vi "LabVIEW Task Manager.vi"() -> ()   [LabVIEW 2010]
doc: "Use this template to create an application that executes until you click the Stop button. Unlike the Single Loop Application VI that uses polling, this VI uses the Event Structure."
uses:
  Error Task_Manager/Error Task_Manager Class/Error Task Manager.lvclass
panel:
  in  "error in (no error)":errorcluster
  in  "Search Clones Up To":i32=100 min=0 step=1
  in  "Timeout (ms)":i32=2000
  in  "Globals?":bool=TRUE
  in  "vit & ctt":bool=TRUE
  in  "Exclude vi.lib?":bool=TRUE
  in  "vi":bool
  in  "ctl":bool=TRUE
  in  "Refresh":bool
  in  "App Instance:":u16(ring) items=["Default Application Instance", "Task Manager.lvproj:My Computer"]
  in  "Data Tree":string[](tree)=["Get File Extension.vi"]
  in  "Close Front Panel":bool
  in  "Toggle Pause":bool
  in  "Pause Source":string
  in  "Initialize":bool
  in  "Close Block Diagram":bool
  in  "Pause":bool
  in  "Resume":bool
  in  "Toggle ExecHilite":bool
  in  "Open Front Panel":bool
  in  "Open Block Diagram":bool
  in  "Abort":bool
  # "Filter"
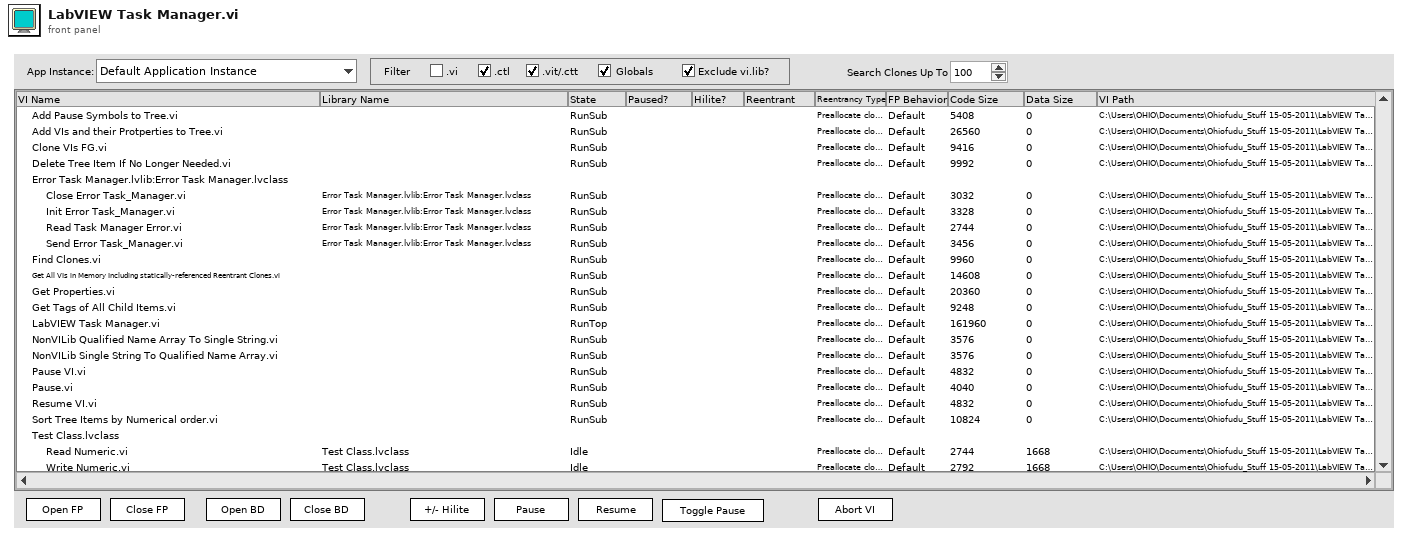
[diagram p1: front panel]
types:
  T1 = cluster{"Sort Column":i32, "Sorted AZ?":bool, "Data Tree Ref":refnum<vi>, "FP Ref":refnum<vi>, "Column Data Type":enum16{"String", "Numeric"}[], "AppInst":refnum<vi>}
  T2 = enum32{"Bad", "Idle", "Run top level", "Running"}
  T3 = typedef "LVPoint32TypeDef.ctl" = cluster{"Horizontal":i32, "Vertical":i32}
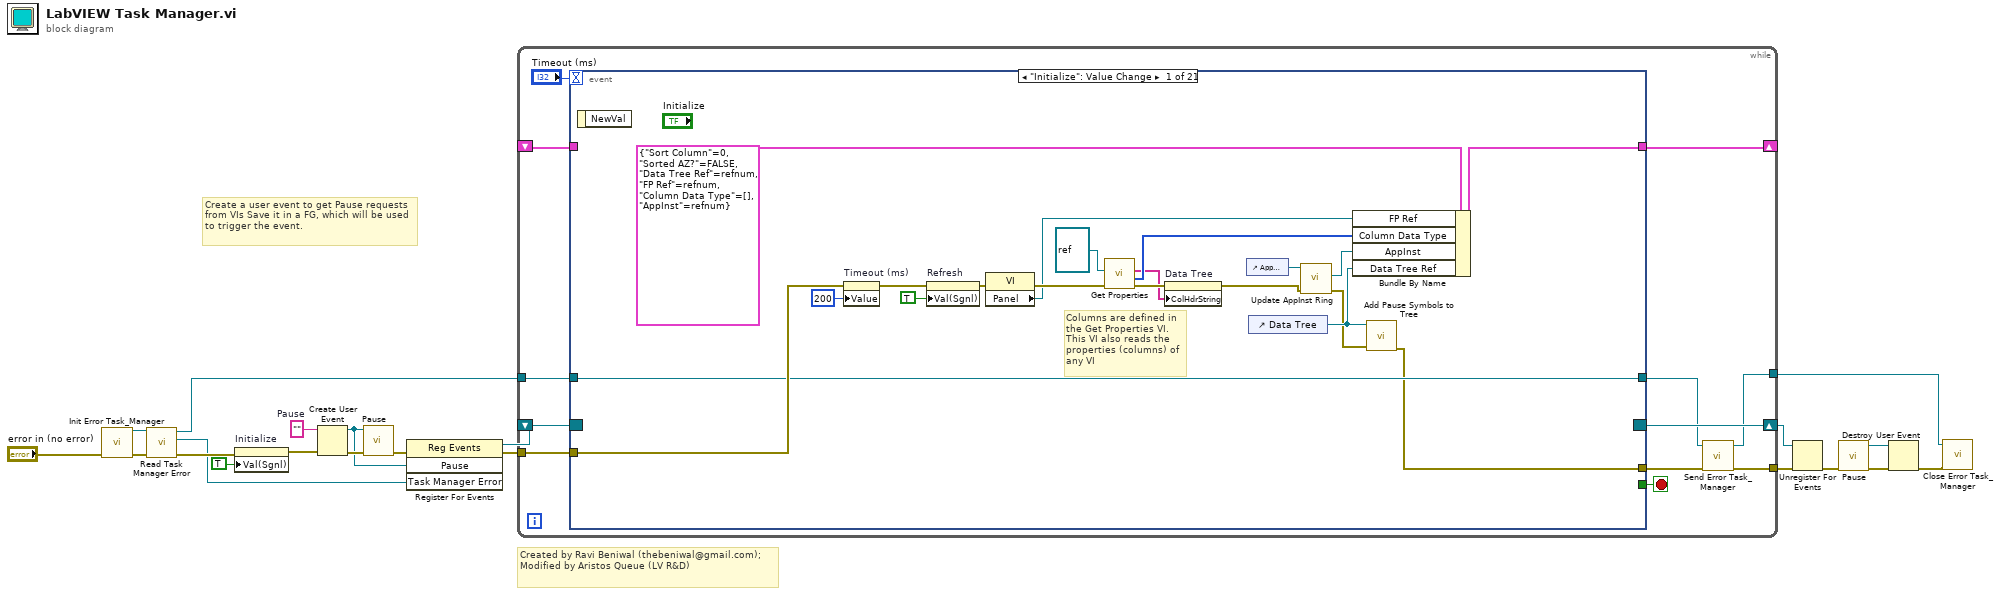
[diagram p0: block diagram]
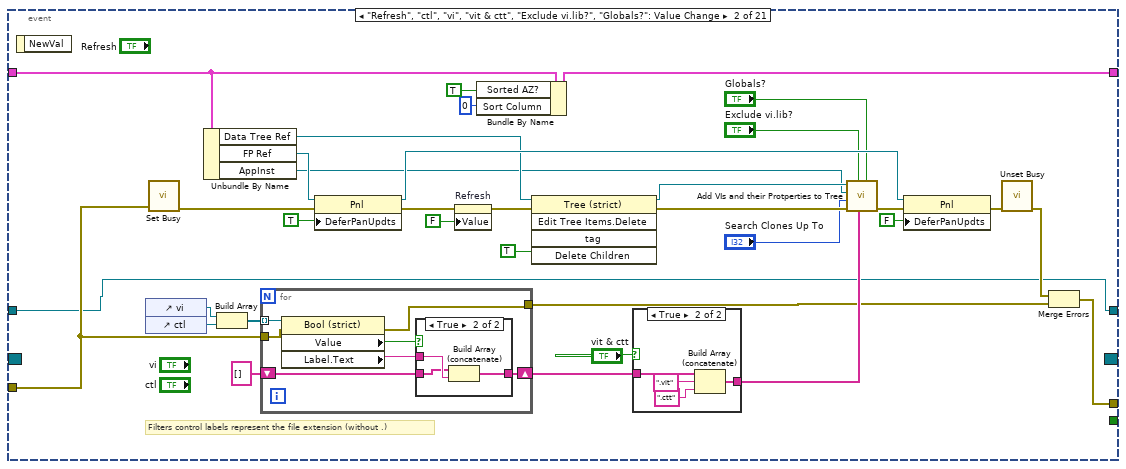
[diagram p2: hidden frame]
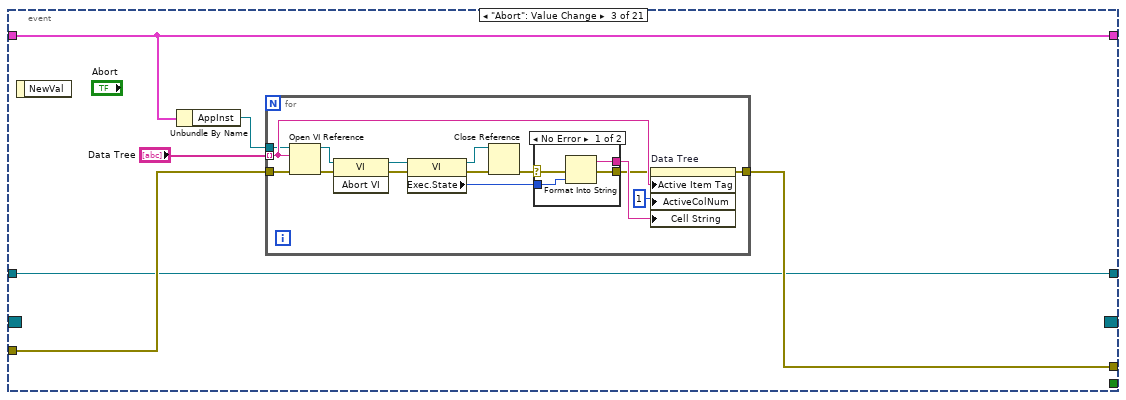
[diagram p5: hidden frame]
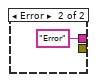
[diagram p6: hidden frame]
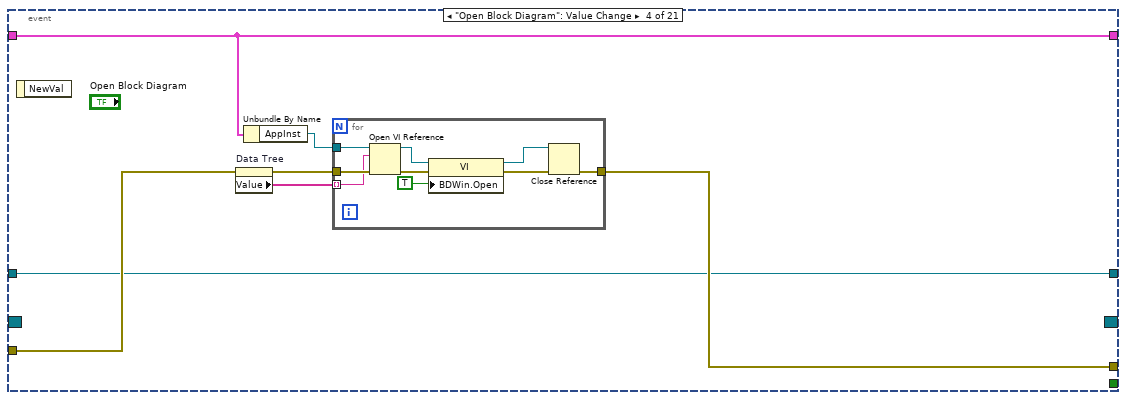
[diagram p7: hidden frame]
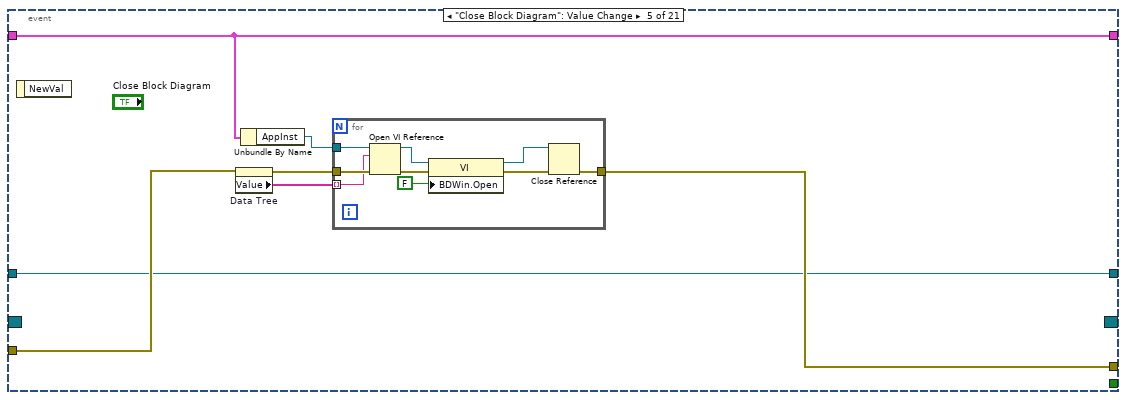
[diagram p8: hidden frame]
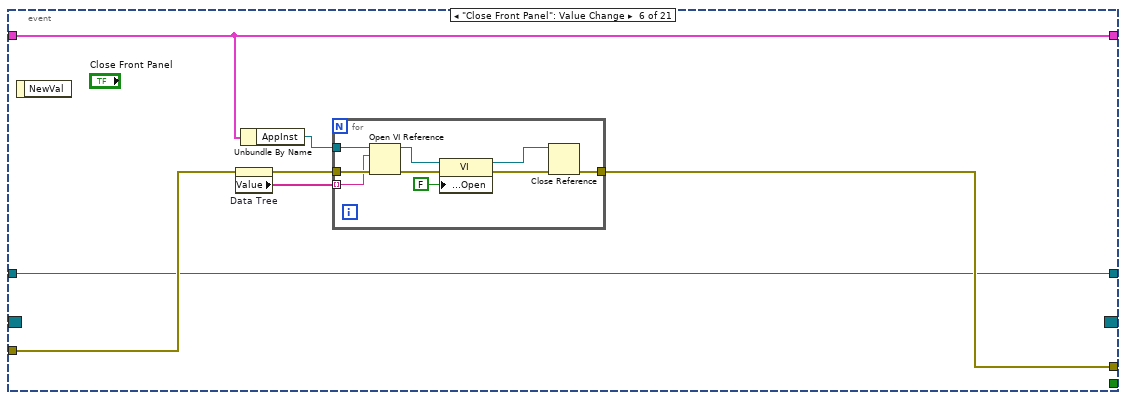
[diagram p9: hidden frame]
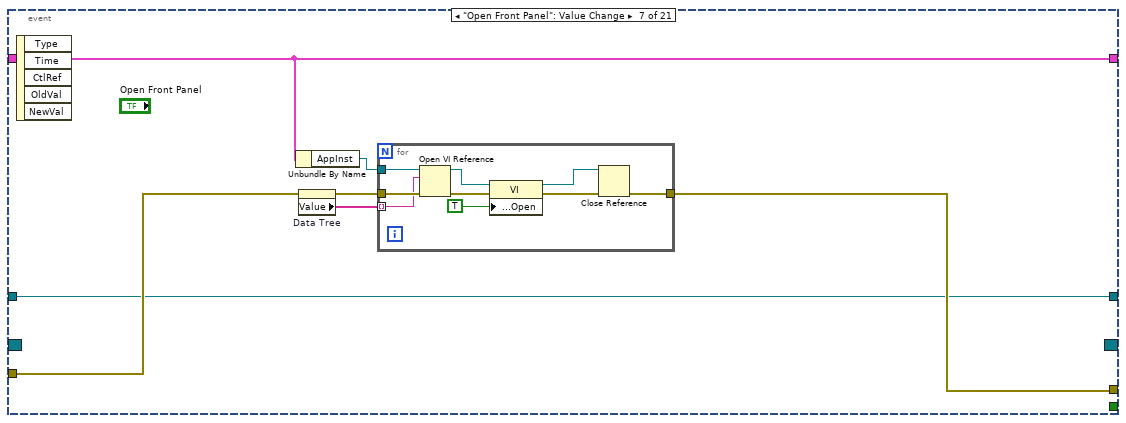
[diagram p10: hidden frame]
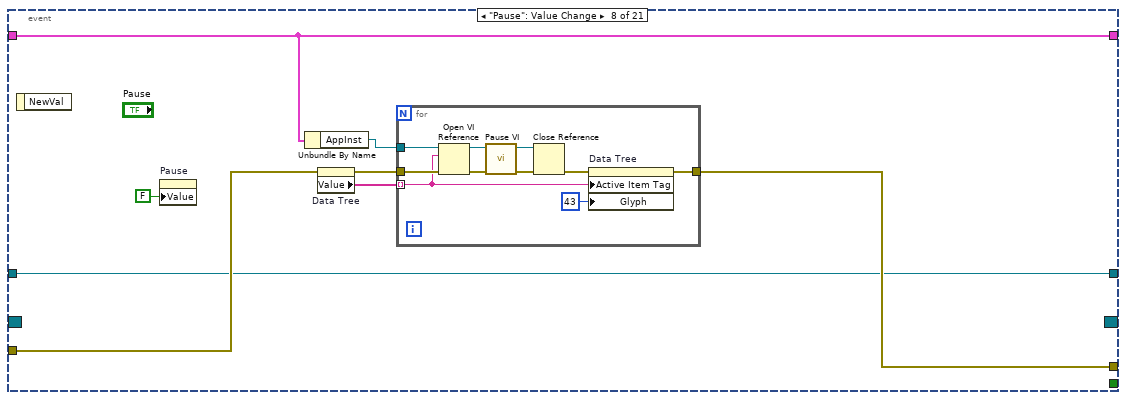
[diagram p11: hidden frame]
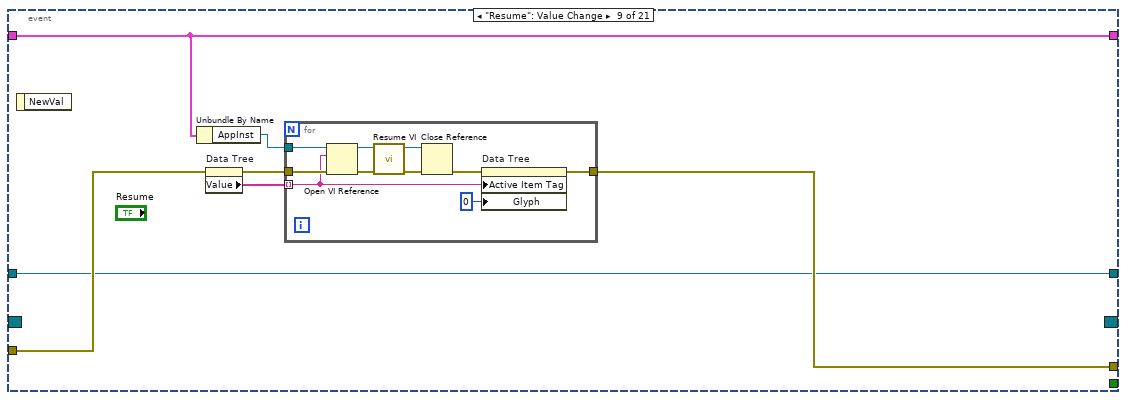
[diagram p12: hidden frame]
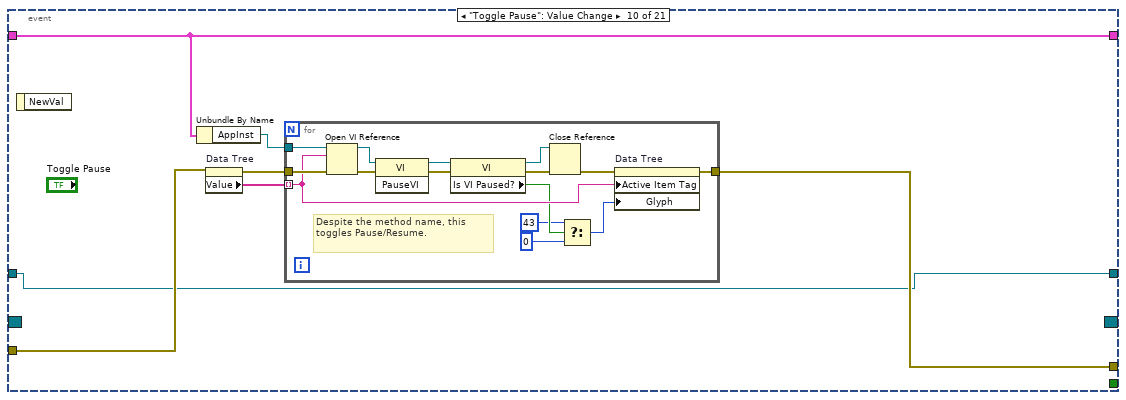
[diagram p13: hidden frame]
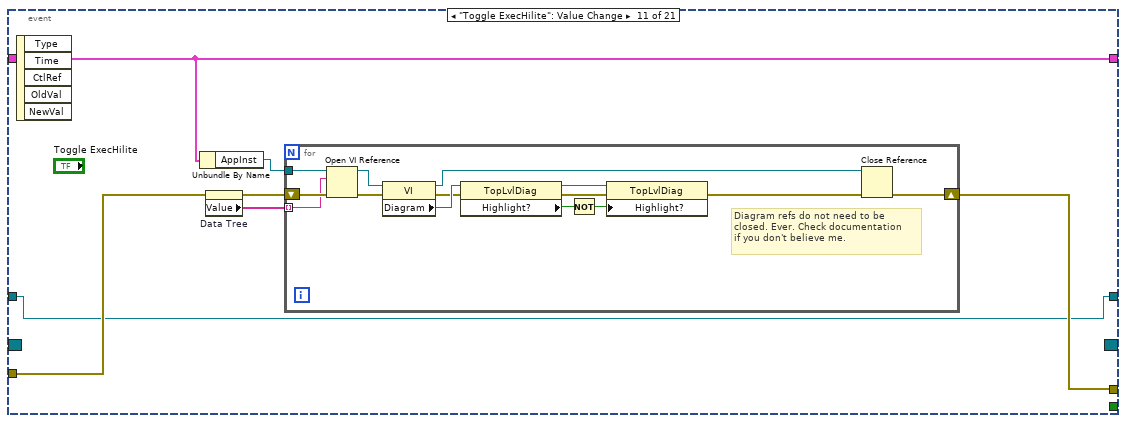
[diagram p14: hidden frame]
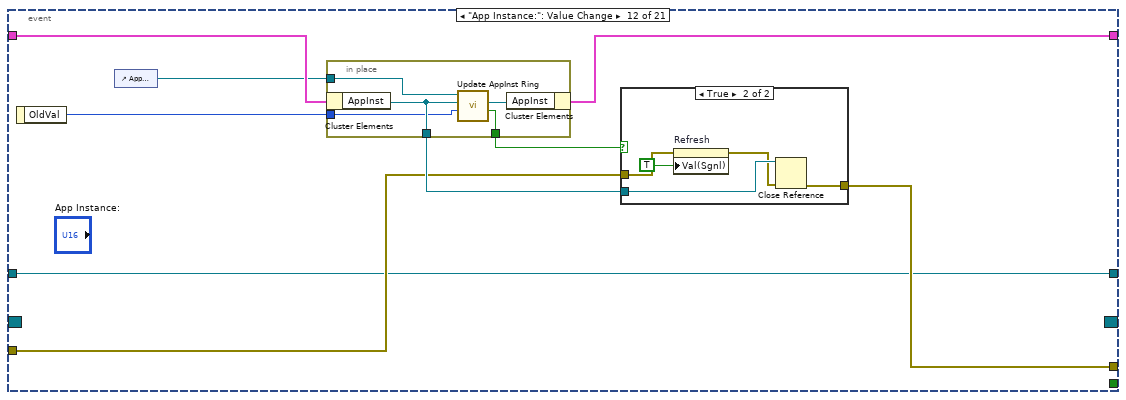
[diagram p15: hidden frame]
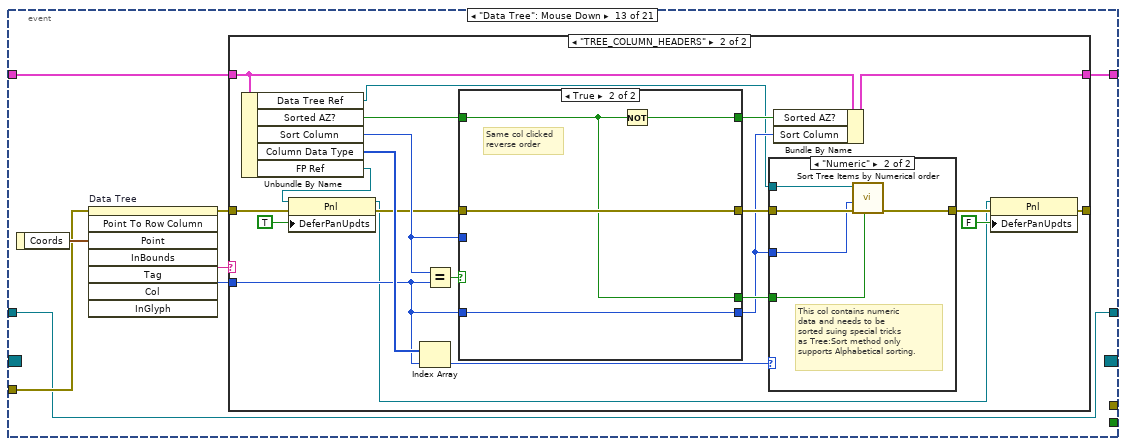
[diagram p17: hidden frame]
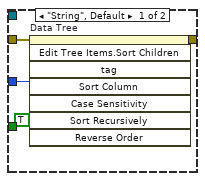
[diagram p19: hidden frame]
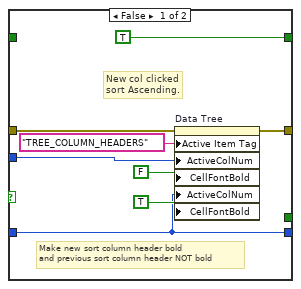
[diagram p20: hidden frame]
diagram:
  w14 = ""  # Pause
  # "Create a user event to get Pause requests from VIs Save it in a FG, which will be used to trigger the event."
  # "Created by Ravi Beniwal (thebeniwal@gmail.com);\nModified by Aristos Queue (LV R&D)"
  n1 = call "Init Error Task_Manager.vi"("error in (no error)"="error in (no error)") -> ("error out"=w6:errorcluster, "Error Task Manager out"=w7:refnum<class "Error Task Manager.lvclass">)  [unwired: 9 in]
  n2 = call "Read Task Manager Error.vi"("error in (no error)"=w6, "Error Task Manager in"=w7) -> ("error out"=w5:errorcluster, "Task Manager Error"=w4:refnum<user-event>, "Error Task Manager out"=w3:refnum<class "Error Task Manager.lvclass">)  [unwired: 7 in]
  n3 = property on="Initialize" class="Bool (strict)"(error in=w5, "Val(Sgnl)"=TRUE ("Value (Signaling)")) -> (error out=w9:errorcluster)  [unwired: 1 in, 1 out]
  n4 = Create User Event(user event datatype=w14, error in=w9) -> (user event=w12:refnum<user-event>, error out=w16:errorcluster)
  n5 = call "Pause.vi"("error in (no error)"=w16, "Pause user event"=w12) -> ("error out"=w15:errorcluster)  [unwired: 8 in, 1 out]
  n6 = register-events(error in=w15, w12, w4) -> (reference out=w13:refnum<event-registration>, error out=w11:errorcluster)  [unwired: 1 in]
  n7 = while {
    shift-right: [w30] -> _
    shift-left: _ -> [w31]
    shift-right: [w29] -> w20
    shift-left: w13 -> [w28]
    tunnel: w11 -> [w27]
    tunnel: [w23] -> w10
    tunnel: w3 -> [w26]
    tunnel: [w22] -> w1
    stop <- w33 stop-if-true
    n8 = event shown="[0] \"Initialize\": Value Change" {
      selector: w28 -> [_ _ _ _ _ _ _ _ _ _ _ _ _ _ _ _ _ _ _ _ _]
      dyn-events: [_ _ _ _ _ _ _ _ _ _ _ _ _ _ _ _ _ _ _ _ _] -> w29
      timeout: "Timeout (ms)" -> [_ _ _ _ _ _ _ _ _ _ _ _ _ _ _ _ _ _ _ _ _]
      tunnel: [_ _ _ _ _ _ _ _ _ _ _ _ _ _ TRUE ("stop") _ w417 _ _ w492 _] -> w33
      tunnel: w31 -> [_ w70 w108 w134 w149 w165 w181 w198 w215 w232 w254 w280 w294 w351 w397 w407 w419 w443 w489 w499 w511]
      tunnel: [w42 w73 w108 w134 w149 w165 w181 w198 w215 w232 w254 w279 w295 w351 w397 w407 w419 w443 w489 w499 w511] -> w30
      tunnel: w27 -> [w38 w58 w106 w132 w148 w164 w180 w196 w214 w231 w253 w274 w293 w347 w396 w402 w416 w430 w486 w491 w504]
      tunnel: [w34 w55 w105 w131 w147 w163 w179 w195 w213 w230 w252 w273 _ w346 w396 w401 w416 w429 w485 w491 w503] -> w24
      tunnel: w26 -> [w35 w54 w104 w130 w146 w162 w178 w194 w212 w229 w251 w272 w292 w345 w395 w400 w415 w428 w484 w490 w502]
      tunnel: [w35 w54 w104 w130 w146 w162 w178 w194 w212 w229 w251 w272 w292 w345 w395 w400 w415 w428 w484 w490 w502] -> w25
      event "Initialize": Value Change {
        # "Columns are defined in the Get Properties VI. This VI also reads the properties (columns) of any VI"
        n9 = event-data() -> ()  [unwired: 2 out]
        n10 = property on="Timeout (ms)" class="DigNum (strict)"(error in=w38, "Value"=200 ("Timeout (ms)")) -> (error out=w40:errorcluster)  [unwired: 1 in, 1 out]
        n11 = property on="Refresh" class="Bool (strict)"(error in=w40, "Val(Sgnl)"=TRUE ("Value (Signaling)")) -> (error out=w48:errorcluster)  [unwired: 1 in, 1 out]
        n12 = property class="VI"(error in=w48) -> (error out=w49:errorcluster, "Panel"=w47:refnum<vi>)  [unwired: 1 in, 1 out]
        n13 = call "Get Properties.vi"("error in"=w49, "AppInst"=refnum<vi> refnum) -> ("error out"=w46:errorcluster, "Column Data Type"=w50:enum16{"String", "Numeric"}[], "Column Labels"=w45:string[])  [unwired: 4 in, 3 out]
        n14 = property on="Data Tree" class="Tree (strict)"(error in=w46, "ColHdrString"=w45) -> (error out=w37:errorcluster)  [unwired: 1 in, 1 out]
        n15 = control-ref of="App Instance:"() -> (w51:refnum<vi>)
        n16 = control-ref of="Data Tree"() -> (w39:refnum<vi>)
        n17 = call "Update AppInst Ring.vi"("error in (no error)"=w37, "Ring in"=w51) -> ("error out"=w36:errorcluster, "AppInst out"=w52:refnum<vi>)  [unwired: 7 in, 1 out]
        n18 = Bundle By Name(cluster=T1 {"Sort Column"=0, "Sorted AZ?"=FALSE, "Data Tree Ref"=refnum, "FP Ref"=refnum, "Column Data Type"=[], "AppInst"=refnum}, "FP Ref"=w47, "Column Data Type"=w50, "AppInst"=w52, "Data Tree Ref"=w39) -> (w42:T1)
        n19 = call "Add Pause Symbols to Tree.vi"("error in"=w36, "Data Tree Ref"=w39) -> ("error out"=w34:errorcluster)  [unwired: 9 in]
      }
      event "Refresh", "ctl", "vi", "vit & ctt", "Exclude vi.lib?", "Globals?": Value Change {
        # "Filters control labels represent the file extension (without .)"
        n20 = event-data() -> ()  [unwired: 2 out]
        n21 = control-ref of="vi"() -> (w78:refnum<vi>)
        n22 = control-ref of="ctl"() -> (w65:refnum<vi>)
        n23 = call <vilib>:"Set Busy.vi"("error in (no error)"=w58) -> ("error out"=w67:errorcluster)  [unwired: 9 in, 1 out]
        n24 = Unbundle By Name(w70) -> ("Data Tree Ref"=w69:refnum<vi>, "FP Ref"=w68:refnum<vi>, "AppInst"=w60:refnum<vi>)
        n25 = Build Array(w78, w65) -> (w77:refnum<vi>[])
        n26 = for {
          tunnel: w77 -> [w99] mode=indexing
          shift-right: [w95] -> w64
          shift-left: string[] [] -> [w96]
          tunnel: w58 -> [w94]
          tunnel: [w93] -> w57
          n27 = property class="Bool (strict)"(reference=w99, error in=w94) -> (error out=w93:errorcluster, "Value"=w98:bool, "Label.Text"=w97:string)  [unwired: 1 out]
          n28 = case shown="True" w98 {
            tunnel: w97 -> [_ w103]
            tunnel: w96 -> [w100 w102]
            tunnel: [w100 w101] -> w95
            frame False {
            }
            frame True {
              n29 = Build Array (concatenate)(w102, w103) -> (w101:string[])
            }
          }
        }
        n30 = property class="Pnl"(reference=w68, error in=w67, "DeferPanUpdts"=TRUE ("Defer Panel Updates")) -> (reference out=w71:refnum<vi>, error out=w80:errorcluster)
        n31 = property on="Refresh" class="Bool (strict)"(error in=w80, "Value"=FALSE ("Refresh")) -> (error out=w84:errorcluster)  [unwired: 1 in, 1 out]
        n32 = Bundle By Name(cluster=w70, "Sorted AZ?"=TRUE, "Sort Column"=0) -> (w73:T1)
        n33 = invoke class="Tree (strict)" method="Edit Tree Items.Delete"(reference=w69, error in=w84, "Delete Children"=TRUE ("Delete Children?")) -> (reference out=w85:refnum<vi>, error out=w86:errorcluster)  [unwired: 2 in, 3 out]
        n34 = case shown="True" "vit & ctt" {
          tunnel: w64 -> [w88 w92]
          tunnel: [w88 w89] -> w62
          frame False {
          }
          frame True {
            n35 = Build Array (concatenate)(w92, ".vit", ".ctt") -> (w89:string[])
          }
        }
        n36 = call "Add VIs and their Protperties to Tree.vi"("Globals?"="Globals?", "File Extension Filters"=w62, "Exclude vi.lib?"="Exclude vi.lib?", "error in"=w86, "Search Clones Up To"="Search Clones Up To", "AppInst"=w60, "Data Tree"=w85) -> ("error out"=w72:errorcluster)  [unwired: 4 in]
        n37 = property class="Pnl"(reference=w71, error in=w72, "DeferPanUpdts"=FALSE ("Defer Panel Updates")) -> (error out=w79:errorcluster)  [unwired: 1 out]
        n38 = call <vilib>:"Unset Busy.vi"("error in (no error)"=w79) -> ("error out"=w56:errorcluster)  [unwired: 10 in]
        n39 = Merge Errors(w56, w57) -> (w55:errorcluster)
      }
      event "Abort": Value Change {
        n40 = event-data() -> ()  [unwired: 2 out]
        n41 = Unbundle By Name(w108) -> ("AppInst"=w107:refnum<vi>)
        n42 = for {
          tunnel: [w119] -> w105
          tunnel: "Data Tree" -> [w117] mode=indexing
          tunnel: w107 -> [w111]
          tunnel: w106 -> [w110]
          n43 = Open VI Reference(application reference (local)=w111, vi path=w117, error in (no error)=w110) -> (vi reference=w123:refnum<vi>, error out=w124:errorcluster)  [unwired: 3 out]
          n44 = invoke class="VI" method="Abort VI"(reference=w123, error in=w124) -> (reference out=w121:refnum<vi>, error out=w112:errorcluster)  [unwired: 1 in, 1 out]
          n45 = property class="VI"(reference=w121, error in=w112) -> (reference out=w120:refnum<vi>, error out=w115:errorcluster, "Exec.State"=w122:T2)
          n46 = Close Reference(reference=w120, error in (no error)=w115) -> (error out=w113:errorcluster)
          n47 = case shown="No Error" w113 {
            selector: w113 -> [w125 _]
            tunnel: w122 -> [w128 _]
            tunnel: [w127 "Error"] -> w118
            tunnel: [w126 _] -> w114
            frame No Error {
              n48 = Format Into String(error in=w125, w128) -> (resulting string=w127:string, error out=w126:errorcluster)  [unwired: 2 in]
            }
            frame Error {
            }
          }
          n49 = property on="Data Tree" class="Tree (strict)"(error in=w114, "Active Item Tag"=w117, "ActiveColNum"=1 ("Active Cell:Active Column Number"), "Cell String"=w118) -> (error out=w119:errorcluster)  [unwired: 1 in, 1 out]
        }
      }
      event "Open Block Diagram": Value Change {
        n50 = event-data() -> ()  [unwired: 2 out]
        n51 = property on="Data Tree" class="Tree (strict)"(error in=w132) -> (error out=w136:errorcluster, "Value"=w135:string[])  [unwired: 1 in, 1 out]
        n52 = Unbundle By Name(w134) -> ("AppInst"=w133:refnum<vi>)
        n53 = for {
          tunnel: [w145] -> w131
          tunnel: w136 -> [w144]
          tunnel: w135 -> [w143] mode=indexing
          tunnel: w133 -> [w137]
          n54 = Open VI Reference(application reference (local)=w137, vi path=w143, error in (no error)=w144) -> (vi reference=w141:refnum<vi>, error out=w142:errorcluster)  [unwired: 3 out]
          n55 = property class="VI"(reference=w141, error in=w142, "BDWin.Open"=TRUE ("Block Diagram Window:Open")) -> (reference out=w140:refnum<vi>, error out=w139:errorcluster)
          n56 = Close Reference(reference=w140, error in (no error)=w139) -> (error out=w145:errorcluster)
        }
      }
      event "Close Block Diagram": Value Change {
        n57 = event-data() -> ()  [unwired: 2 out]
        n58 = property on="Data Tree" class="Tree (strict)"(error in=w148) -> (error out=w152:errorcluster, "Value"=w151:string[])  [unwired: 1 in, 1 out]
        n59 = Unbundle By Name(w149) -> ("AppInst"=w150:refnum<vi>)
        n60 = for {
          tunnel: [w161] -> w147
          tunnel: w152 -> [w160]
          tunnel: w151 -> [w159] mode=indexing
          tunnel: w150 -> [w153]
          n61 = Open VI Reference(application reference (local)=w153, vi path=w159, error in (no error)=w160) -> (vi reference=w157:refnum<vi>, error out=w158:errorcluster)  [unwired: 3 out]
          n62 = property class="VI"(reference=w157, error in=w158, "BDWin.Open"=FALSE ("Block Diagram Window:Open")) -> (reference out=w156:refnum<vi>, error out=w155:errorcluster)
          n63 = Close Reference(reference=w156, error in (no error)=w155) -> (error out=w161:errorcluster)
        }
      }
      event "Close Front Panel": Value Change {
        n64 = event-data() -> ()  [unwired: 2 out]
        n65 = property on="Data Tree" class="Tree (strict)"(error in=w164) -> (error out=w168:errorcluster, "Value"=w167:string[])  [unwired: 1 in, 1 out]
        n66 = Unbundle By Name(w165) -> ("AppInst"=w166:refnum<vi>)
        n67 = for {
          tunnel: [w177] -> w163
          tunnel: w168 -> [w176]
          tunnel: w167 -> [w175] mode=indexing
          tunnel: w166 -> [w169]
          n68 = Open VI Reference(application reference (local)=w169, vi path=w175, error in (no error)=w176) -> (vi reference=w173:refnum<vi>, error out=w174:errorcluster)  [unwired: 3 out]
          n69 = property class="VI"(reference=w173, error in=w174, "Front Panel.Open"=FALSE ("Block Diagram Window:Open")) -> (reference out=w172:refnum<vi>, error out=w171:errorcluster)
          n70 = Close Reference(reference=w172, error in (no error)=w171) -> (error out=w177:errorcluster)
        }
      }
      event "Open Front Panel": Value Change {
        n71 = event-data() -> ()  [unwired: 6 out]
        n72 = Unbundle By Name(w181) -> ("AppInst"=w182:refnum<vi>)
        n73 = property on="Data Tree" class="Tree (strict)"(error in=w180) -> (error out=w184:errorcluster, "Value"=w183:string[])  [unwired: 1 in, 1 out]
        n74 = for {
          tunnel: [w193] -> w179
          tunnel: w184 -> [w192]
          tunnel: w183 -> [w191] mode=indexing
          tunnel: w182 -> [w185]
          n75 = Open VI Reference(application reference (local)=w185, vi path=w191, error in (no error)=w192) -> (vi reference=w189:refnum<vi>, error out=w190:errorcluster)  [unwired: 3 out]
          n76 = property class="VI"(reference=w189, error in=w190, "Front Panel.Open"=TRUE ("Block Diagram Window:Open")) -> (reference out=w188:refnum<vi>, error out=w187:errorcluster)
          n77 = Close Reference(reference=w188, error in (no error)=w187) -> (error out=w193:errorcluster)
        }
      }
      event "Pause": Value Change {
        n78 = event-data() -> ()  [unwired: 2 out]
        n79 = property on="Pause" class="Bool (strict)"("Value"=FALSE ("Pause")) -> ()  [unwired: 2 in, 2 out]
        n80 = Unbundle By Name(w198) -> ("AppInst"=w199:refnum<vi>)
        n81 = property on="Data Tree" class="Tree (strict)"(error in=w196) -> (error out=w200:errorcluster, "Value"=w201:string[])  [unwired: 1 in, 1 out]
        n82 = for {
          tunnel: w201 -> [w204] mode=indexing
          tunnel: w200 -> [w207]
          tunnel: [w205] -> w195
          tunnel: w199 -> [w202]
          n83 = Open VI Reference(application reference (local)=w202, vi path=w204, error in (no error)=w207) -> (vi reference=w210:refnum<vi>, error out=w211:errorcluster)  [unwired: 3 out]
          n84 = call "Pause VI.vi"("error in (no error)"=w211, "VI in"=w210) -> ("error out"=w208:errorcluster, "VI out"=w209:refnum<vi>)  [unwired: 8 in]
          n85 = Close Reference(reference=w209, error in (no error)=w208) -> (error out=w206:errorcluster)
          n86 = property on="Data Tree" class="Tree (strict)"(error in=w206, "Active Item Tag"=w204, "Glyph"=43 ("Active Item:Symbol Index")) -> (error out=w205:errorcluster)  [unwired: 1 in, 1 out]
        }
      }
      event "Resume": Value Change {
        n87 = event-data() -> ()  [unwired: 2 out]
        n88 = Unbundle By Name(w215) -> ("AppInst"=w216:refnum<vi>)
        n89 = property on="Data Tree" class="Tree (strict)"(error in=w214) -> (error out=w217:errorcluster, "Value"=w218:string[])  [unwired: 1 in, 1 out]
        n90 = for {
          tunnel: w218 -> [w220] mode=indexing
          tunnel: w217 -> [w224]
          tunnel: [w221] -> w213
          tunnel: w216 -> [w219]
          n91 = Open VI Reference(application reference (local)=w219, vi path=w220, error in (no error)=w224) -> (vi reference=w227:refnum<vi>, error out=w228:errorcluster)  [unwired: 3 out]
          n92 = call "Resume VI.vi"("error in (no error)"=w228, "VI in"=w227) -> ("error out"=w225:errorcluster, "VI out"=w226:refnum<vi>)  [unwired: 8 in]
          n93 = Close Reference(reference=w226, error in (no error)=w225) -> (error out=w222:errorcluster)
          n94 = property on="Data Tree" class="Tree (strict)"(error in=w222, "Active Item Tag"=w220, "Glyph"=0 ("Active Item:Symbol Index")) -> (error out=w221:errorcluster)  [unwired: 1 in, 1 out]
        }
      }
      event "Toggle Pause": Value Change {
        n95 = event-data() -> ()  [unwired: 2 out]
        n96 = Unbundle By Name(w232) -> ("AppInst"=w233:refnum<vi>)
        n97 = property on="Data Tree" class="Tree (strict)"(error in=w231) -> (error out=w234:errorcluster, "Value"=w235:string[])  [unwired: 1 in, 1 out]
        n98 = for {
          tunnel: w235 -> [w247] mode=indexing
          tunnel: w234 -> [w250]
          tunnel: [w248] -> w230
          tunnel: w233 -> [w246]
          # "Despite the method name, this\ntoggles Pause/Resume."
          n99 = Open VI Reference(application reference (local)=w246, vi path=w247, error in (no error)=w250) -> (vi reference=w244:refnum<vi>, error out=w245:errorcluster)  [unwired: 3 out]
          n100 = invoke class="VI" method="PauseVI"(reference=w244, error in=w245) -> (reference out=w243:refnum<vi>, error out=w242:errorcluster)  [unwired: 1 in, 1 out]
          n101 = property class="VI"(reference=w243, error in=w242) -> (reference out=w240:refnum<vi>, error out=w241:errorcluster, "Is VI Paused?"=w239:bool)
          n102 = Close Reference(reference=w240, error in (no error)=w241) -> (error out=w249:errorcluster)
          n103 = Select(t=43, s=w239, f=0 ("Active Item:Symbol Index")) -> (s? t:f=w236:i32)
          n104 = property on="Data Tree" class="Tree (strict)"(error in=w249, "Active Item Tag"=w247, "Glyph"=w236) -> (error out=w248:errorcluster)  [unwired: 1 in, 1 out]
        }
      }
      event "Toggle ExecHilite": Value Change {
        n105 = event-data() -> ()  [unwired: 6 out]
        n106 = Unbundle By Name(w254) -> ("AppInst"=w255:refnum<vi>)
        n107 = property on="Data Tree" class="Tree (strict)"(error in=w253) -> (error out=w257:errorcluster, "Value"=w256:string[])  [unwired: 1 in, 1 out]
        n108 = for {
          tunnel: w256 -> [w269] mode=indexing
          shift-right: [w271] -> w252
          shift-left: w257 -> [w270]
          tunnel: w255 -> [w258]
          # "Diagram refs do not need to be\nclosed. Ever. Check documentation\nif you don't believe me."
          n109 = Open VI Reference(application reference (local)=w258, vi path=w269, error in (no error)=w270) -> (vi reference=w267:refnum<vi>, error out=w268:errorcluster)  [unwired: 3 out]
          n110 = property class="VI"(reference=w267, error in=w268) -> (reference out=w266:refnum<vi>, error out=w262:errorcluster, "Diagram"=w265:refnum<vi>)
          n111 = property class="TopLvlDiag"(reference=w265, error in=w262) -> (reference out=w259:refnum<vi>, error out=w261:errorcluster, "Highlight?"=w263:bool)
          n112 = Not(x=w263) -> (.not. x?=w264:bool)
          n113 = property class="TopLvlDiag"(reference=w259, error in=w261, "Highlight?"=w264) -> (error out=w260:errorcluster)  [unwired: 1 out]
          n114 = Close Reference(reference=w266, error in (no error)=w260) -> (error out=w271:errorcluster)
        }
      }
      event "App Instance:": Value Change {
        n115 = event-data() -> ("OldVal"=w275:u16)  [unwired: 1 out]
        n116 = control-ref of="App Instance:"() -> (w278:refnum<vi>)
        n117 = in-place {
          in-place-border: w278 -> [w290]
          in-place-border: [w289] -> w277
          in-place-border: [w288] -> w276
          in-place-border: w275 -> [w287]
          n118 = in-place-cluster #1(w280) -> ("AppInst"=w288:refnum<vi>)
          n119 = call "Update AppInst Ring.vi"("Old Value"=w287, "AppInst in"=w288, "Ring in"=w290) -> ("Selection Changed?"=w289:bool, "AppInst out"=w291:refnum<vi>)  [unwired: 6 in, 1 out]
          n120 = in-place-cluster #1("AppInst"=w291) -> (w279:T1)
        }
        n121 = case shown="True" w277 {
          tunnel: w276 -> [_ w285]
          tunnel: w274 -> [w281 w284]
          tunnel: [w281 w282] -> w273
          frame False {
          }
          frame True {
            n122 = property on="Refresh" class="Bool (strict)"(error in=w284, "Val(Sgnl)"=TRUE ("Value (Signaling)")) -> (error out=w283:errorcluster)  [unwired: 1 in, 1 out]
            n123 = Close Reference(reference=w285, error in (no error)=w283) -> (error out=w282:errorcluster)
          }
        }
      }
      event "Data Tree": Mouse Down {
        n124 = event-data() -> ("Coords"=w299:T3)  [unwired: 1 out]
        n125 = invoke on="Data Tree" class="Tree (strict)" method="Point To Row Column"(error in=w293, "Point"=w299) -> (error out=w297:errorcluster, "Tag"=w298:string, "Col"=w296:i32)  [unwired: 6 in, 5 out]
        n126 = case shown="\"TREE_COLUMN_HEADERS\"" w298 {
          tunnel: w297 -> [w301 w308]
          tunnel: w296 -> [_ w312]
          tunnel: [w301 w303] -> _
          tunnel: [w300 w321] -> w295
          tunnel: w294 -> [w300 w322]
          frame Default {
          }
          frame "TREE_COLUMN_HEADERS" {
            n127 = Unbundle By Name(w322) -> ("Data Tree Ref"=w310:refnum<vi>, "Sorted AZ?"=w319:bool, "Sort Column"=w314:i32, "Column Data Type"=w313:enum16{"String", "Numeric"}[], "FP Ref"=w306:refnum<vi>)
            n128 = property class="Pnl"(reference=w306, error in=w308, "DeferPanUpdts"=TRUE ("Defer Panel Updates")) -> (reference out=w302:refnum<vi>, error out=w307:errorcluster)
            n129 = Index Array(array=w313, index=w312) -> (element=w311:enum16{"String", "Numeric"})
            n130 = Equal?(x=w314, y=w312) -> (x = y?=w320:bool)
            n131 = case shown="True" w320 {
              tunnel: w319 -> [_ w342]
              tunnel: [TRUE ("Sorted AZ?") w341] -> w318
              tunnel: [_ w342] -> w317
              tunnel: w307 -> [w336 w344]
              tunnel: [w335 w344] -> w316
              tunnel: w312 -> [w334 w343]
              tunnel: [w334 w343] -> w315
              tunnel: w314 -> [w333 _]
              frame False {
                # "Make new sort column header bold\nand previous sort column header NOT bold"
                # "New col clicked\nsort Ascending."
                n132 = property on="Data Tree" class="Tree (strict)"(error in=w336, "Active Item Tag"="TREE_COLUMN_HEADERS" ("Active Item:Tag"), "ActiveColNum"=w333, "CellFontBold"=FALSE ("Active Cell:Cell Font:Bold"), "ActiveColNum"=w334, "CellFontBold"=TRUE ("Active Cell:Cell Font:Bold")) -> (error out=w335:errorcluster)  [unwired: 1 in, 1 out]
              }
              frame True {
                # "Same col clicked\nreverse order"
                n133 = Not(x=w342) -> (.not. x?=w341:bool)
              }
            }
            n134 = case shown="\"Numeric\"" w311 {
              tunnel: [w327 w331] -> w304
              tunnel: w317 -> [w326 w330]
              tunnel: w316 -> [w325 w332]
              tunnel: w315 -> [w324 w328]
              tunnel: w310 -> [_ w329]
              frame "String", Default {
                n135 = invoke on="Data Tree" class="Tree (strict)" method="Edit Tree Items.Sort Children"(error in=w325, "Sort Column"=w324, "Sort Recursively"=TRUE ("Sort Recursively?"), "Reverse Order"=w326) -> (error out=w327:errorcluster)  [unwired: 4 in, 7 out]
              }
              frame "Numeric" {
                # "This col contains numeric\ndata and needs to be\nsorted suing special tricks\nas Tree:Sort method only\nsupports Alphabetical sorting."
                n136 = call "Sort Tree Items by Numerical order.vi"("Reverse Order?"=w330, "error in"=w332, "Sort Column"=w328, "Data Tree"=w329) -> ("error out"=w331:errorcluster)  [unwired: 7 in]
              }
            }
            n137 = Bundle By Name(cluster=w322, "Sorted AZ?"=w318, "Sort Column"=w315) -> (w321:T1)
            n138 = property class="Pnl"(reference=w302, error in=w304, "DeferPanUpdts"=FALSE ("Defer Panel Updates")) -> (error out=w303:errorcluster)  [unwired: 1 out]
          }
        }
      }
      event Timeout {
        # "Not all the properties will change between consecutive runs of this case, but it was just quicker and easier to code and maintain it this way."
        n139 = event-data() -> ()  [unwired: 3 out]
        n140 = Unbundle By Name(w351) -> ("Data Tree Ref"=w348:refnum<vi>, "Column Data Type"=w356:enum16{"String", "Numeric"}[], "Sort Column"=w355:i32, "Sorted AZ?"=w354:bool, "FP Ref"=w358:refnum<vi>, "AppInst"=w350:refnum<vi>)
        n141 = property class="Pnl"(reference=w358, error in=w347, "DeferPanUpdts"=TRUE ("Defer Panel Updates")) -> (reference out=w359:refnum<vi>, error out=w360:errorcluster)
        n142 = Index Array(array=w356, index=w355) -> (element=w353:enum16{"String", "Numeric"})
        n143 = property on="Data Tree" class="Tree (strict)"(error in=w360) -> (error out=w364:errorcluster, "All Tags"=w363:string[])  [unwired: 1 in, 1 out]
        n144 = for {
          tunnel: w364 -> [w381]
          tunnel: w363 -> [w380] mode=indexing
          tunnel: [w377] -> w349
          tunnel: w350 -> [w376]
          tunnel: w348 -> [w374]
          n145 = call "Get Properties.vi"("error in"=w381, "AppInst"=w376, "VI Name"=w380) -> ("error out"=w375:errorcluster, "Full Name Out"=w379:string, "VI Properties"=w378:string[])  [unwired: 3 in, 3 out]
          n146 = case shown="No Error" w375 {
            selector: w375 -> [w382 _]
            tunnel: w379 -> [w386 w394]
            tunnel: w378 -> [w384 _]
            tunnel: [w383 w393] -> w377
            tunnel: w374 -> [_ w392]
            frame No Error {
              n147 = property on="Data Tree" class="Tree (strict)"(error in=w382, "Active Item Tag"=w386) -> (error out=w385:errorcluster)  [unwired: 1 in, 1 out]
              n148 = for {
                tunnel: w385 -> [w391]
                tunnel: w384 -> [w388] mode=indexing
                tunnel: [w387] -> w383
                i -> [w390]
                n149 = Increment(x=w390) -> (x+1=w389:i32)
                n150 = property on="Data Tree" class="Tree (strict)"(error in=w391, "ActiveColNum"=w389, "Cell String"=w388) -> (error out=w387:errorcluster)  [unwired: 1 in, 1 out]
              }
            }
            frame Error {
              n151 = call "Delete Tree Item If No Longer Needed.vi"("Item Tag"=w394, "Tree Ref"=w392) -> ("error out"=w393:errorcluster)  [unwired: 9 in]
            }
          }
        }
        n152 = Not(x=w354) -> (.not. x?=w352:bool)
        n153 = case shown="\"Numeric\"" w353 {
          tunnel: [w368 w372] -> w357
          tunnel: w352 -> [w367 w371]
          tunnel: w349 -> [w366 w373]
          tunnel: w355 -> [w365 w369]
          tunnel: w348 -> [_ w370]
          frame "String", Default {
            n154 = invoke on="Data Tree" class="Tree (strict)" method="Edit Tree Items.Sort Children"(error in=w366, "Sort Column"=w365, "Reverse Order"=w367) -> (error out=w368:errorcluster)  [unwired: 5 in, 7 out]
          }
          frame "Numeric" {
            # "This col contains numeric\ndata and needs to be\nsorted suing special tricks\nas Tree:Sort method only\nsupports Alphabetical sorting."
            n155 = call "Sort Tree Items by Numerical order.vi"("Reverse Order?"=w371, "error in"=w373, "Sort Column"=w369, "Data Tree"=w370) -> ("error out"=w372:errorcluster)  [unwired: 7 in]
          }
        }
        n156 = property class="Pnl"(reference=w359, error in=w357, "DeferPanUpdts"=FALSE ("Defer Panel Updates")) -> (error out=w346:errorcluster)  [unwired: 1 out]
      }
      event Panel Close? {
        n157 = event-data() -> ()  [unwired: 2 out]
        n158 = event-data("Discard?"=TRUE) -> ()  [unwired: 1 in, 1 out]
      }
      event Menu Activation? {
        n159 = event-data() -> ("MenuRef"=w406:refnum<k9>)  [unwired: 1 out]
        n160 = property on="Timeout (ms)" class="DigNum (strict)"() -> ("Value"=w403:i32)  [unwired: 2 in, 2 out]
        n161 = for {
          tunnel: w406 -> [w414]
          tunnel: string[] ["Paused", "High", "Normal", "Low"] -> [w413] mode=indexing
          tunnel: w403 -> [w412]
          tunnel: i32[] [-1, 200, 1000, 5000] -> [w410] mode=indexing
          tunnel: w402 -> [w409]
          tunnel: [w408] -> w401
          n162 = Equal?(x=w410, y=w412) -> (x = y?=w411:bool)
          n163 = Set Menu Item Info(6:w411, 7:w413, 8:w409, 11:w414) -> (0:w408:errorcluster)  [unwired: 3 in, 1 out]
        }
        n164 = event-data() -> ()  [unwired: 2 in, 1 out]
      }
      event Menu Selection (User) {
        n165 = event-data() -> ("ItemTag"=w418:string)  [unwired: 1 out]
        n166 = case shown="\"High\", \"Low\", \"Normal\", \"Paused\"" w418 {
          selector: w418 -> [_ _ w421 _]
          tunnel: [_ TRUE ("stop") _ _] -> w417
          frame Default {
          }
          frame "Exit" {
          }
          frame "High", "Low", "Normal", "Paused" {
            n167 = case shown="\"Normal\", Default" w421 {
              tunnel: [5000 ("Value (Signaling)") 1000 ("Value (Signaling)") 200 ("Value (Signaling)") -1 ("Value (Signaling)")] -> w422
              frame "Low" {
              }
              frame "Normal", Default {
              }
              frame "High" {
              }
              frame "Paused" {
              }
            }
            n168 = property on="Timeout (ms)" class="DigNum (strict)"("Val(Sgnl)"=w422) -> ()  [unwired: 2 in, 2 out]
          }
          frame "Refresh Now" {
            n169 = property on="Refresh" class="Bool (strict)"("Val(Sgnl)"=TRUE ("Value (Signaling)")) -> ()  [unwired: 2 in, 2 out]
          }
        }
      }
      event User Event {
        # "If this is a Clone, mark it as the source of the pause event"
        # "Call Pause event case\nto pause selected VIs"
        n170 = event-data() -> ("Pause"=w431:string)  [unwired: 1 out]
        n171 = Unbundle By Name(w443) -> ("AppInst"=w442:refnum<vi>)
        n172 = Open VI Reference(application reference (local)=w442, vi path=w431, error in (no error)=w430) -> (vi reference=w441:refnum<vi>, error out=w440:errorcluster)  [unwired: 3 out]
        n173 = property class="VI"(reference=w441, error in=w440) -> (reference out=w438:refnum<vi>, error out=w439:errorcluster, "IsCloneVI"=w432:bool)
        n174 = Close Reference(reference=w438, error in (no error)=w439) -> (error out=w434:errorcluster)
        n175 = case shown="True" w432 {
          tunnel: w431 -> [w448 w456]
          tunnel: [w449 w450] -> w437
          tunnel: w434 -> [_ _]
          frame False {
            n176 = Build Array(w448) -> (w449:string[])
          }
          frame True {
            # "VI that generated the Pause is a clone. Select all clones of the original VI."
            n177 = property on="Data Tree" class="Tree (strict)"() -> ("All Tags"=w451:string[])  [unwired: 2 in, 2 out]
            n178 = Search/Split String(string=w456, search string/char (-)=":") -> (substring before match=w452:string)  [unwired: 1 in, 2 out]
            n179 = for {
              shift-right: [w465] -> w454
              shift-left: w451 -> [w466]
              tunnel: w451 -> [w461] mode=indexing
              shift-right: [w464] -> w453
              shift-left: 0 -> [w463]
              tunnel: w452 -> [w458]
              n180 = Search/Split String(string=w461, search string/char (-)=":") -> (substring before match=w459:string, offset of match=w460:i32)  [unwired: 1 in, 1 out]
              n181 = case shown="0, Default" w460 {
                tunnel: w466 -> [w474 w483]
                tunnel: [w473 w483] -> w465
                tunnel: [w472 w482] -> w464
                tunnel: w463 -> [w471 w482]
                tunnel: w461 -> [w470 _]
                tunnel: w459 -> [w469 _]
                tunnel: w458 -> [w468 _]
                frame 0, Default {
                  n182 = Equal?(x=w468, y=w469) -> (x = y?=w467:bool)
                  n183 = case shown="True" w467 {
                    tunnel: w474 -> [w479 w481]
                    tunnel: [w476 w481] -> w473
                    tunnel: [w477 w480] -> w472
                    tunnel: w471 -> [w478 w480]
                    tunnel: w470 -> [w475 _]
                    frame True {
                      n184 = Increment(x=w478) -> (x+1=w477:i32)
                      n185 = Replace Array Subset(array=w479, new element=w475, index=w478) -> (w476:string[])
                    }
                    frame False {
                    }
                  }
                }
                frame -1 {
                }
              }
            }
            n186 = Array Subset(array=w454, length=w453) -> (w450:string[])  [unwired: 1 in]
          }
        }
        n187 = property on="Data Tree" class="Tree (strict)"("Value"=w437) -> (error out=w435:errorcluster)  [unwired: 2 in, 1 out]
        n188 = property on="Pause" class="Bool (strict)"(error in=w435, "Val(Sgnl)"=TRUE ("Value (Signaling)")) -> (error out=w433:errorcluster)  [unwired: 1 in, 1 out]
        n189 = case shown="False" w432 {
          tunnel: w433 -> [w444 w447]
          tunnel: w431 -> [_ w446]
          tunnel: [w444 w445] -> w429
          frame False {
          }
          frame True {
            n190 = property on="Pause Source" class="Str"(error in=w447, "Val(Sgnl)"=w446) -> (error out=w445:errorcluster)  [unwired: 1 in, 1 out]
          }
        }
      }
      event "Pause Source": Value Change {
        n191 = event-data() -> ("NewVal"=w487:string)  [unwired: 1 out]
        n192 = property on="Data Tree" class="Tree (strict)"(error in=w486, "Active Item Tag"=w487, "Glyph"=44 ("Active Item:Symbol Index")) -> (error out=w485:errorcluster)  [unwired: 1 in, 1 out]
      }
      event User Event {
        n193 = event-data() -> ("source"=w496:string)  [unwired: 1 out]
        n194 = Concatenate Strings("!!Error Task Manager !!" ("string"), w496) -> (w494:string)
        n195 = Two Button Dialog(message=w494, 1:"Ignore Error" ("F button name (\"Cancel\")"), 2:"End Task Manager" ("T button name (\"OK\")")) -> (T button?=w493:bool)
        n196 = case shown="False" w493 {
          selector: w493 -> [w500 w501]
          tunnel: [w500 w501] -> w492
          frame False {
          }
          frame True {
          }
        }
      }
      event "Data Tree": Double Click {
        n197 = event-data() -> ("Tag"=w513:string)  [unwired: 1 out]
        n198 = Unbundle By Name(w511) -> ("AppInst"=w512:refnum<vi>)
        n199 = Open VI Reference(application reference (local)=w512, vi path=w513, error in (no error)=w504) -> (vi reference=w515:refnum<vi>, error out=w514:errorcluster)  [unwired: 3 out]
        n200 = property class="VI"(reference=w515, error in=w514) -> (reference out=w507:refnum<vi>, error out=w508:errorcluster, "BDWin.Open"=w510:bool, "Front Panel.Open"=w509:bool)
        n201 = case shown="False" w510 {
          selector: w510 -> [_ w531]
          tunnel: w508 -> [w519 w532]
          tunnel: w509 -> [w520 _]
          tunnel: w507 -> [w518 w530]
          tunnel: [w517 w529] -> w506
          tunnel: [w516 w528] -> w505
          frame False {
            n202 = case shown="True" w520 {
              selector: w520 -> [_ w527]
              tunnel: w519 -> [w521 w526]
              tunnel: w518 -> [w522 w525]
              tunnel: [w522 w524] -> w517
              tunnel: [w521 w523] -> w516
              frame False {
              }
              frame True {
                n203 = property class="VI"(reference=w525, error in=w526, "Front Panel.Open"=w527) -> (reference out=w524:refnum<vi>, error out=w523:errorcluster)
              }
            }
          }
          frame True {
            # "Bring window to front"
            n204 = property class="VI"(reference=w530, error in=w532, "BDWin.Open"=w531) -> (reference out=w529:refnum<vi>, error out=w528:errorcluster)
          }
        }
        n205 = Close Reference(reference=w506, error in (no error)=w505) -> (error out=w503:errorcluster)
      }
    }
    n206 = call "Send Error Task_Manager.vi"("error in (no error)"=w24, "Error Task Manager in"=w25) -> ("error out"=w23:errorcluster, "Error Task Manager out"=w22:refnum<class "Error Task Manager.lvclass">)  [unwired: 8 in]
  }
  n207 = Unregister For Events(event registration refnum=w20, error in=w10) -> (error out=w19:errorcluster)
  n208 = call "Pause.vi"("error in (no error)"=w19) -> ("error out"=w18:errorcluster, "user event Out"=w17:refnum<user-event>)  [unwired: 9 in]
  n209 = Destroy User Event(user event=w17, error in=w18) -> (error out=w2:errorcluster)
  n210 = call "Close Error Task_Manager.vi"("error in (no error)"=w2, "Error Task Manager in"=w1) -> ()  [unwired: 9 in, 1 out]
